vi "Read.vi"(5 "Number of channels to read":i32=1, 7 "signal id":i32=1, 8 "error in":errorcluster, 9 "tiemout [s]":dbl=1.5, 10 "Samples count":i32=1, 11 "MicroDAQ.lvlib:DSP.lvclass":refnum<class "DSP.lvclass">) -> (0 "error out":errorcluster, 2 "data":dbl[][](array[numeric]), 3 "MicroDAQ.lvlib:DSP.lvclass out":refnum<class "DSP.lvclass">)   [LabVIEW 2009, in "MicroDAQ.lvlib" / "DSP.lvclass"]
uses:
  <instrlib>/MicroDAQ/Channel/DSP/DSP.lvclass
  <instrlib>/MicroDAQ/Channel/Channel.lvclass
  <instrlib>/MicroDAQ/Mlink library wraper/mlink.lvlib
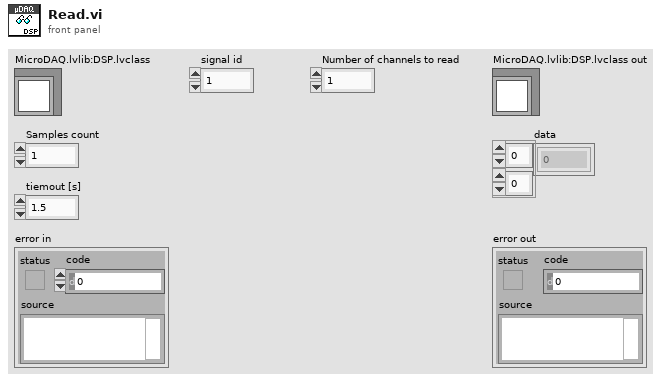
[diagram p1: front panel]
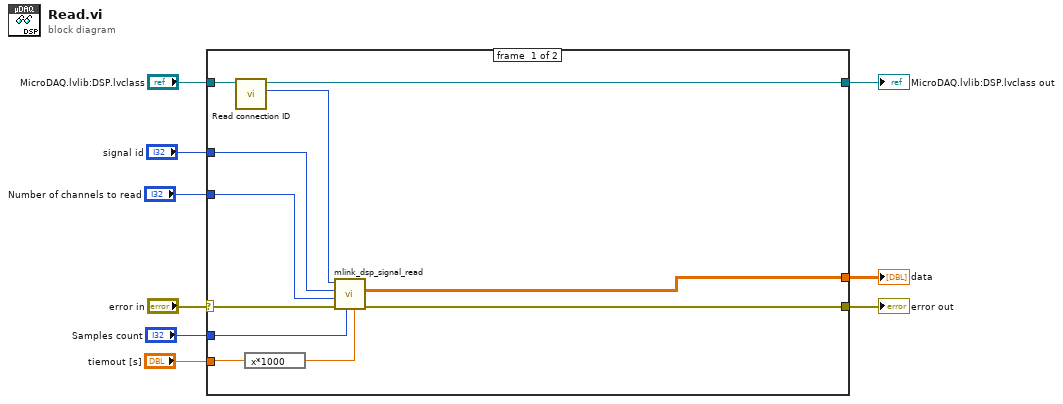
[diagram p0: block diagram]
diagram:
  n1 = case shown="No Error" "error in" {
    selector: "error in" -> [w18 w21]
    tunnel: "MicroDAQ.lvlib:DSP.lvclass" -> [w20 w22]
    tunnel: [w17 w21] -> w8
    tunnel: [w19 w22] -> w6
    tunnel: "signal id" -> [w15 _]
    tunnel: "Number of channels to read" -> [w14 _]
    tunnel: "Samples count" -> [w13 _]
    tunnel: "tiemout [s]" -> [w11 _]
    tunnel: [w12 _] -> w1
    frame #0 {
      n2 = call <instrlib>:"Read connection ID.vi"("Task in"=w20) -> ("connection ID"=w16:i32, "Task out"=w19:refnum<class "DSP.lvclass">)  [unwired: 9 in]
      n3 = expression code="x*1000"(w11) -> (w10:dbl)
      n4 = call <instrlib>:"mlink_dsp_signal_read.vi"("tiemout"=w10, "count"=w13, "error in (no error)"=w18, "signal size"=w14, "signal ID"=w15, "connection ID"=w16) -> ("error out"=w17:errorcluster, "data out"=w12:dbl[][])  [unwired: 3 in, 1 out]
    }
    frame #1 {
    }
  }
  "error out" <- w8
  "MicroDAQ.lvlib:DSP.lvclass out" <- w6
  "data" <- w1
